vi "1L07-num-vers-nb_decimales.vi"(11 "nombre":dbl) -> (3 "nb dec.":i32)   [LabVIEW 2010, in "lv_01.lvlib"]
uses:
  lv_01.lvlib
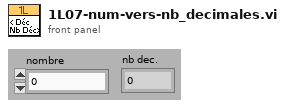
[diagram p1: front panel]
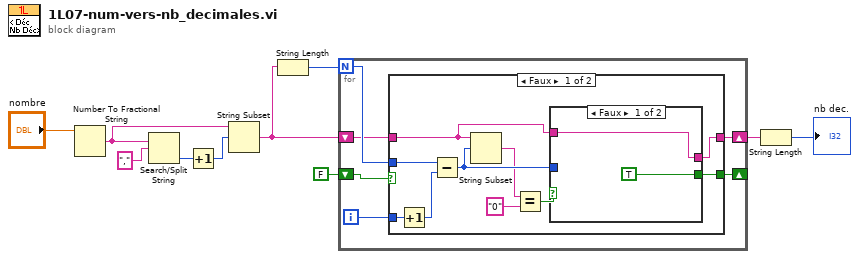
[diagram p0: block diagram]
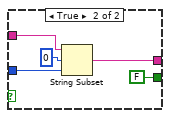
[diagram p2: hidden frame]
diagram:
  n1 = Number To Fractional String(number="nombre") -> (F-format string=w8:string)  [unwired: 3 in]
  n2 = Search/Split String(string=w8, search string/char (-)="," ("chaîne/car. recherché (-)")) -> (offset of match=w7:i32)  [unwired: 1 in, 2 out]
  n3 = Increment(x=w7) -> (x+1=w6:i32)
  n4 = String Subset(string=w8, offset (0)=w6) -> (substring=w4:string)  [unwired: 1 in]
  n5 = String Length(string=w4) -> (length=w5:i32)
  n6 = for {
    N: w5 -> [w16]
    shift-right: [w14] -> w2
    shift-left: w4 -> [w13]
    shift-right: [w12] -> _
    shift-left: FALSE -> [w11]
    i -> [w15]
    n7 = case shown="Faux" w11 {
      selector: w11 -> [_ w35]
      tunnel: w16 -> [w26 _]
      tunnel: w15 -> [w25 _]
      tunnel: [w22 w34] -> w14
      tunnel: w13 -> [w18 w34]
      tunnel: [w20 w35] -> w12
      frame False {
        n8 = Increment(x=w25) -> (x+1=w23:i32)
        n9 = Subtract(x=w26, y=w23) -> (x-y=w19:i32)
        n10 = String Subset(string=w18, offset (0)=w19) -> (substring=w17:string)  [unwired: 1 in]
        n11 = Equal?(x=w17, y="0") -> (x = y?=w21:bool)
        n12 = case shown="Faux" w21 {
          tunnel: w18 -> [w28 w33]
          tunnel: w19 -> [_ w30]
          tunnel: [w28 w32] -> w22
          tunnel: [TRUE FALSE] -> w20
          frame False {
          }
          frame True {
            n13 = String Subset(string=w33, offset (0)=0, length (rest)=w30) -> (substring=w32:string)
          }
        }
      }
      frame True {
      }
    }
  }
  n14 = String Length(string=w2) -> (length=→"nb dec.":i32)
